vi "SunCluster.vi"() -> (0 "XY Sun Cluster":cluster{dbl[], dbl[]})   [LabVIEW 2020]
doc: "Returns cluster with information about Sun's position."
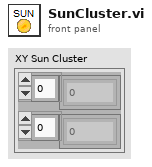
[diagram p1: front panel]
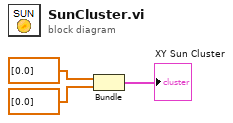
[diagram p0: block diagram]
diagram:
  n1 = Bundle(dbl[] [0.0], dbl[] [0.0]) -> (→"XY Sun Cluster":cluster{dbl[], dbl[]})  [unwired: 1 in]
